vi "TPV FPGA.vi"() -> ()   [LabVIEW 2019]
uses:
  <vilib>/eio/EIONode/EIONode.xnode
  <vilib>/rvi/eio/common/nirviEmuTemplateMethod_errors.vi
  <vilib>/rvi/DataTransferAndStorage/Container/XNode/niFpgaContainer.xnode
  <vilib>/rvi/interface/RandomDataEmulation/nirviRandomDataFpgaReadWriteTemplate.vi
panel:
  out "Overflow":bool
  in  "Count(mSec)":u32
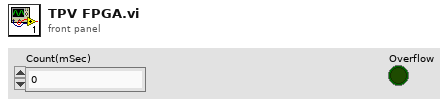
[diagram p1: front panel]
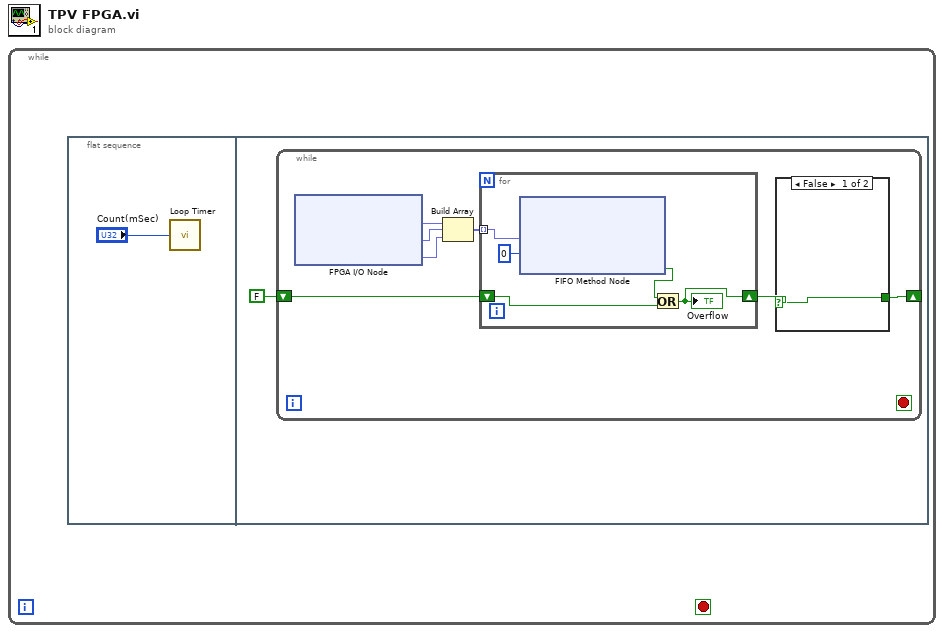
[diagram p0: block diagram]
diagram:
  n1 = while {
    stop <- _ stop-if-true
    n2 = flat-sequence {
      frame #0 {
        n3 = call "Loop Timer"("Count(mSec)"="Count(mSec)") -> ()  [unwired: 1 out]
      }
      frame #1 {
        n4 = while {
          shift-right: [w3] -> _
          shift-left: FALSE ("y") -> [w5]
          stop <- _ stop-if-true
          n5 = xnode "FPGA I/O Node"() -> ("Mod1/TC0"=w9:fxp<+/-,24,-2>, "Mod1/Autozero"=w8:fxp<+/-,24,-2>, "Mod1/CJC"=w7:fxp<+/-,24,-2>)  [unwired: 3 in, 3 out]
          n6 = Build Array(w9, w8, w7) -> (w6:fxp<+/-,24,-2>[])
          n7 = for {
            tunnel: w6 -> [w15] mode=indexing
            shift-right: [w11] -> w4
            shift-left: w5 -> [w12]
            n8 = xnode ("FIFO Method Node")("Element"=w15, "Timeout"=0) -> ("Timed Out?"=w13:bool)  [unwired: 1 in, 1 out]
            n9 = Or(x=w13, y=w12) -> (x .or. y?=w11:bool)
            "Overflow" <- w11
          }
          n10 = case shown="False" w4 {
            selector: w4 -> [w10 _]
            tunnel: [w10 _] -> w3
            frame False {
            }
            frame True {
            }
          }
        }
      }
    }
  }
